vi "Pretank Carl M.vi"() -> ()   [LabVIEW 2018]
panel:
  out "Boolean":bool
  in  "Temp preset Value":dbl
  in  "Tank Preset Value":dbl
  in  "Reset":bool
  in  "?":bool
  out "Status":string
  out "Cup Filling":bool
  out "Temperture":dbl(slide) scale=0.0..100.0
  out "TANK":dbl(slide) scale=0.0..10.0
  in  "Heat Tank":dbl
  in  "Fill Tank":dbl
  in  "Sensor 2":bool
  in  "Sensor 1":bool
  out "Heater ON":bool
  out "Conveyor ON":bool
  out "Pump ON":bool
  in  "Start":bool
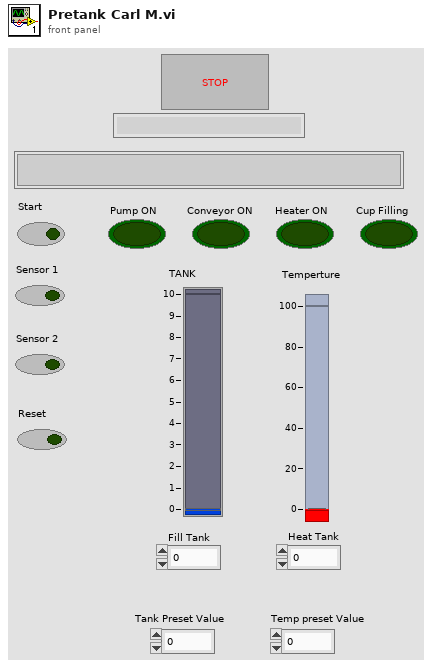
[diagram p1: front panel]
types:
  T1 = enum16{"Start", "Fill", "Sensor 1", "Heat", "Cup", "Sensor 2", "OFF"}
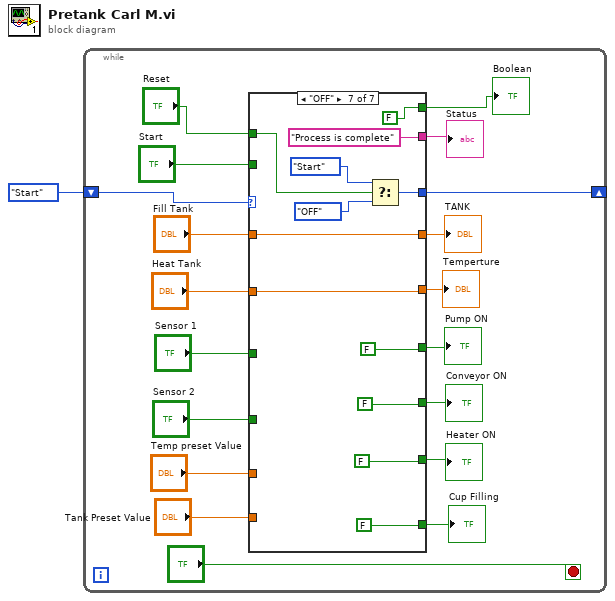
[diagram p0: block diagram]
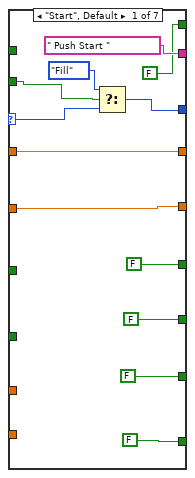
[diagram p2: hidden frame]
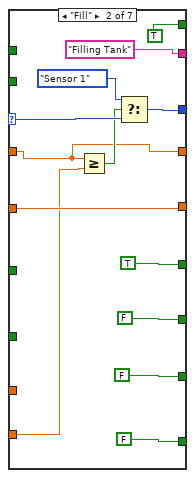
[diagram p3: hidden frame]
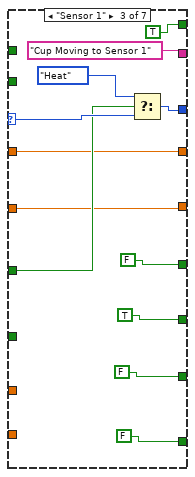
[diagram p4: hidden frame]
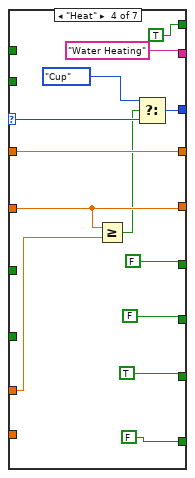
[diagram p5: hidden frame]
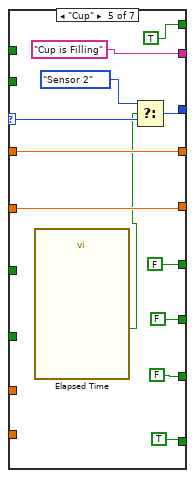
[diagram p6: hidden frame]
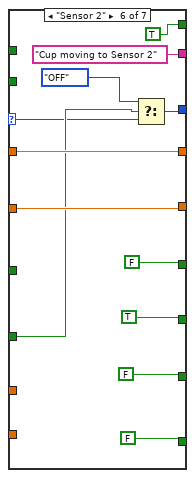
[diagram p7: hidden frame]
diagram:
  n1 = while {
    shift-right: [w17] -> _
    shift-left: T1."Start" -> [w19]
    stop <- "?" stop-if-true
    n2 = case shown="\"OFF\"" w19 {
      selector: w19 -> [w29 w43 w55 w68 w74 w84 _]
      tunnel: [" Push Start " "Filling Tank" "Cup Moving to Sensor 1" "Water Heating" "Cup is Filling" "Cup moving to Sensor 2" "Process is complete"] -> w18
      tunnel: [w30 w44 w56 w67 w79 w92 w96] -> w17
      tunnel: "Fill Tank" -> [w28 w41 w48 w69 w78 w91 w106]
      tunnel: [w28 w41 w48 w69 w78 w91 w106] -> w15
      tunnel: "Heat Tank" -> [w27 w40 w47 w61 w77 w90 w105]
      tunnel: [w27 w40 w47 w61 w77 w90 w105] -> w13
      tunnel: "Sensor 2" -> [_ _ _ _ _ w85 _]
      tunnel: "Sensor 1" -> [_ _ w49 _ _ _ _]
      tunnel: [FALSE TRUE FALSE FALSE FALSE FALSE FALSE] -> w10
      tunnel: [FALSE FALSE TRUE FALSE FALSE TRUE FALSE] -> w9
      tunnel: [FALSE FALSE FALSE TRUE FALSE FALSE FALSE] -> w8
      tunnel: [FALSE FALSE FALSE FALSE TRUE FALSE FALSE] -> w7
      tunnel: "Start" -> [w22 _ _ _ _ _ _]
      tunnel: "Reset" -> [_ _ _ _ _ _ w97]
      tunnel: "Temp preset Value" -> [_ _ _ w59 _ _ _]
      tunnel: "Tank Preset Value" -> [_ w34 _ _ _ _ _]
      tunnel: [FALSE TRUE TRUE TRUE TRUE TRUE FALSE] -> w2
      frame "Start", Default {
        n3 = Select(t=T1."Fill", s=w22, f=w29) -> (s? t:f=w30:T1)
      }
      frame "Fill" {
        n4 = Greater Or Equal?(x=w41, y=w34) -> (x >= y?=w42:bool)
        n5 = Select(t=T1."Sensor 1", s=w42, f=w43) -> (s? t:f=w44:T1)
      }
      frame "Sensor 1" {
        n6 = Select(t=T1."Heat", s=w49, f=w55) -> (s? t:f=w56:T1)
      }
      frame "Heat" {
        n7 = Greater Or Equal?(x=w61, y=w59) -> (x >= y?=w60:bool)
        n8 = Select(t=T1."Cup", s=w60, f=w68) -> (s? t:f=w67:T1)
      }
      frame "Cup" {
        n9 = call "Elapsed Time"() -> ("Time has Elapsed"=w72:bool)  [unwired: 12 in, 7 out]
        n10 = Select(t=T1."Sensor 2", s=w72, f=w74) -> (s? t:f=w79:T1)
      }
      frame "Sensor 2" {
        n11 = Select(t=T1."OFF", s=w85, f=w84) -> (s? t:f=w92:T1)
      }
      frame "OFF" {
        n12 = Select(t=T1."Start", s=w97, f=T1."OFF") -> (s? t:f=w96:T1)
      }
    }
    "Pump ON" <- w10
    "Conveyor ON" <- w9
    "Heater ON" <- w8
    "TANK" <- w15
    "Temperture" <- w13
    "Cup Filling" <- w7
    "Status" <- w18
    "Boolean" <- w2
  }
